vi "main.vi"() -> ()   [LabVIEW 2019]
uses:
  LabJackU3/temperature_status_LabJackU3.ctl
  MKS946/cluster_ref_MKS946.ctl
  MaxiGauge/cluster_ref_MaxiGauge.ctl
  Fridge_Valve/cluster_ref_fridge_valve.ctl
  BGA244/cluster_ref_BGA244.ctl
  TPG361/cluster_ref_TPG361.ctl
  MCC_ETC/cluster_ref_MCCETC.ctl
  MKS670/cluster_ref_MKS670.ctl
  LabJackU3/cluster_ref_LabJackU3.ctl
  ITM10/cluster_ref_ITM10.ctl
  THCD_401/cluster_ref_thcd401.ctl
  Magnet_PS/cluster_ref_MagPS.ctl
  LakeShore218/cluster_ref_LakeShore218.ctl
  RootsPumpLCW/cluster_ref_RootsPumpLCW.ctl
  THCD_400/thcd_controls/variable_reference.ctl
panel:
  out "level_fridge_LHe":dbl(slide) caption="%" scale=0.0..45.0 scale format="%#.1f"
  out "level_fridge_LN2":dbl(slide) caption="%" scale=0.0..100.0 scale format="%#.1f"
  out "MCCETC02_T7":dbl caption="Sep. Line" format="%.1f"
  in  "open_RPLCW":bool caption="open_THCD_400"
  out "RPLCW_WFS1":dbl caption="WFS1" format="%.1f"
  out "RPLCW_M4":dbl caption="M4" format="%.1f"
  out "RPLCW_M3":dbl caption="M3" format="%.1f"
  out "PRLCW_M2":dbl caption="M2" format="%.1f"
  out "RPLCW_M1":dbl caption="M1" format="%.1f"
  out "RPLCW_status":bool
  in  "open_LS218_02":bool caption="open_THCD_400"
  out "LS218_02_T7":dbl format="%.1f"
  out "LS218_02_T6":dbl format="%.1f"
  out "LS218_02_T5":dbl format="%.1f"
  out "LS218_02_T4":dbl format="%.1f"
  out "LS218_02_T3":dbl caption="W" format="%.1f"
  out "LS218_02_T2":dbl format="%.1f"
  out "LS218_02_T1":dbl caption="W" format="%.1f"
  out "LS218_02_status":bool
  out "Nose LHe Level":dbl(slide) caption="%" scale=0.0..100.0 scale format="%#_1f"
  in  "open_MagPS":bool caption="open_THCD_400"
  out "MagPS_status":bool
  out "LS218_01_T8":dbl caption="W" format="%.1f"
  out "LS218_01_T7":dbl caption="W" format="%.1f"
  out "LS218_01_T6":dbl caption="W" format="%.1f"
  out "LS218_01_T5":dbl caption="W" format="%.1f"
  out "LS218_01_T4":dbl caption="W" format="%.1f"
  out "LS218_01_T3":dbl caption="W" format="%.1f"
  out "LS218_01_T2":dbl caption="W" format="%.1f"
  out "LS218_01_T1":dbl caption="W" format="%.1f"
  out "THCD401_status":bool
  out "FC1":dbl format="%.2f"
  out "FC2":dbl format="%.2f"
  out "FM1":dbl format="%.2f"
  in  "open_THCD_401":bool caption="open_THCD_400"
  out "MCCETC03_T5":dbl format="%.1f"
  out "MCCETC03_T4":dbl format="%.1f"
  in  "open_ITM10":bool caption="open_THCD_400"
  out "T_Coil_B":dbl caption="Coil B" format="%.1f"
  out "T_Coil_T":dbl caption="Coil T" format="%.1f"
  out "T_Tank_B":dbl caption="Tank B" format="%.1f"
  out "T_Tank_T":dbl caption="Tank T" format="%.1f"
  out "ITM10_status":bool
  out "MG5":dbl caption="psi" format="%.2f"
  in  "open_LJU3_TC":bool caption="open_THCD_400"
  out "LJU3_T_status":T1=enum."UNKNOWN" caption="QT Comp. LCW Temp."
  out "LJU3_TC_status":bool
  out "MKS670_100_status":bool
  out "p_mks670_100":dbl caption="Torr"
  in  "open_LS218_01":bool caption="open_THCD_400"
  out "LS218_01_status":bool
  in  "open_MCCETC03":bool caption="open_THCD_400"
  out "MCCETC03_T3":dbl caption="T3" format="%.1f"
  out "MCCETC03_T2":dbl caption="T2" format="%.1f"
  out "MCCETC03_T1":dbl caption="T1" format="%.1f"
  out "MCCETC03_T0":dbl caption="T0" format="%.1f"
  out "MCCETC03_status":bool
  in  "open_MCCETC01":bool caption="open_THCD_400"
  out "MCCETC01_T7":dbl caption="DR" format="%.1f"
  out "MCCETC01_T6":dbl caption="DL" format="%.1f"
  out "MCCETC01_T5":dbl caption="DB" format="%.1f"
  out "MCCETC01_T4":dbl caption="DT" format="%.1f"
  out "MCCETC01_T3":dbl caption="UR" format="%.1f"
  out "MCCETC01_T2":dbl caption="UL" format="%.1f"
  out "MCCETC01_T1":dbl caption="UB" format="%.1f"
  out "MCCETC01_T0":dbl caption="UT" format="%.1f"
  out "MCCETC01_status":bool
  out "MCCETC02_T6":dbl caption="Sep. Line" format="%.2f"
  out "MCCETC02_T5":dbl caption="LHe FL #2" format="%.1f"
  out "MCCETC02_T4":dbl caption="LHe FL #1" format="%.1f"
  out "MCCETC02_T3":dbl caption="LHe FL Stinger" format="%.1f"
  out "MCCETC02_T2":dbl caption="Fridge Top" format="%.1f"
  in  "open_MCCETC02":bool caption="open_THCD_400"
  out "MCCETC02_T1":dbl caption="IVC Top" format="%.2f"
  out "MCCETC02_T0":dbl caption="IVC Bottom" format="%.2f"
  out "MCCETC02_status":bool
  in  "open_TPG361":bool caption="open_THCD_400"
  out "TPG361_p":dbl caption="IVC" format="%_3e"
  out "TPG361_status":bool
  in  "open_BGA244":bool caption="open_THCD_400"
  out "Purity":dbl caption="%" format="%.2f"
  out "BGA244_status":bool
  out "MKS670_He3_status":bool
  out "MKS670_1000_status":bool
  in  "all_stop_button":bool
  in  "open_MaxiGauge":bool
  out "MG_status":bool
  out "MG4":dbl format="%_4f"
  out "MG3":dbl format="%_4f"
  out "MG2":dbl caption="Torr" format="%_4f"
  out "MG1":dbl caption="Torr" format="%_4f"
  out "Fridge_Valve_status":bool
  in  "open_Fridge_Valve":bool
  in  "open_MKS670_He3":bool
  in  "open_MKS670_100":bool
  in  "open_MKS670_1000":bool
  in  "open_THCD_400":bool
  out "THCD400_status":bool
  out "FC1_400":dbl format="%.2f"
  out "FC2_400":dbl format="%.2f"
  out "FM1_400":dbl caption="Fridge Return" format="%.2f"
  out "Bypass Valve":dbl format="%_3f"
  out "P2":dbl caption="Root Exhaust" format="%.2f"
  out "He3 Vapor Pressure":dbl
  out "MKS946_status":bool
  out "p_mks670_1000":dbl caption="Torr"
  out "Run-Valve":dbl format="%_3f"
  in  "open_MKS946":bool
  out "P1":dbl caption="QT Manifold" format="%.2f"
  in  "STOP VI":bool
  # "THCD-400"
  # "Click a reading and stay for 1 sec to find its controller name."
  # "Fridge Temperatures"
  # "GPM"
  # "Microwave System"
  # "psi"
  # "°C"
  # "L/m"
  # "psi"
  # "Turns"
  # "L/m"
  # "L/m"
  # "°C"
  # "°C"
  # "Controller"
  # "Status"
  # "Sub Panel"
  # "Torr"
  # "Torr"
  # "MKS 670 / 1000"
  # "Cooldown-Line Temp."
  # "°C"
  # "MKS 670 /   100"
  # "K"
  # "MKS 670 / He3"
  # "Turns"
  # "MKS 946"
  # "THCD-401"
  # "°C"
  # "MaxiGauge"
  # "K"
  # "Fridge Valve"
  # "°C"
  # "Target-Cup\nTemperatures"
  # "°C"
  # "K"
  # "BGA244"
  # "TPG361"
  # "°C"
  # "K"
  # "ITM10"
  # "Torr"
  # "W"
  # "MCC E-TC #01"
  # "K"
  # "MCC E-TC #02"
  # "°C"
  # "Torr"
  # "%"
  # "MCC E-TC #03"
  # "K"
  # "LakeShore218 #01"
  # "K"
  # "LakeShore218 #02"
  # "%"
  # "°C"
  # "Roots-Pump LCW"
  # "Magnet Surface Temperature"
  # "LabJack U3 TC"
  # "K"
  # "Magnet PS"
  # "K"
  # "Schematic Version 7.0"
  # "Cryo Control Panel"
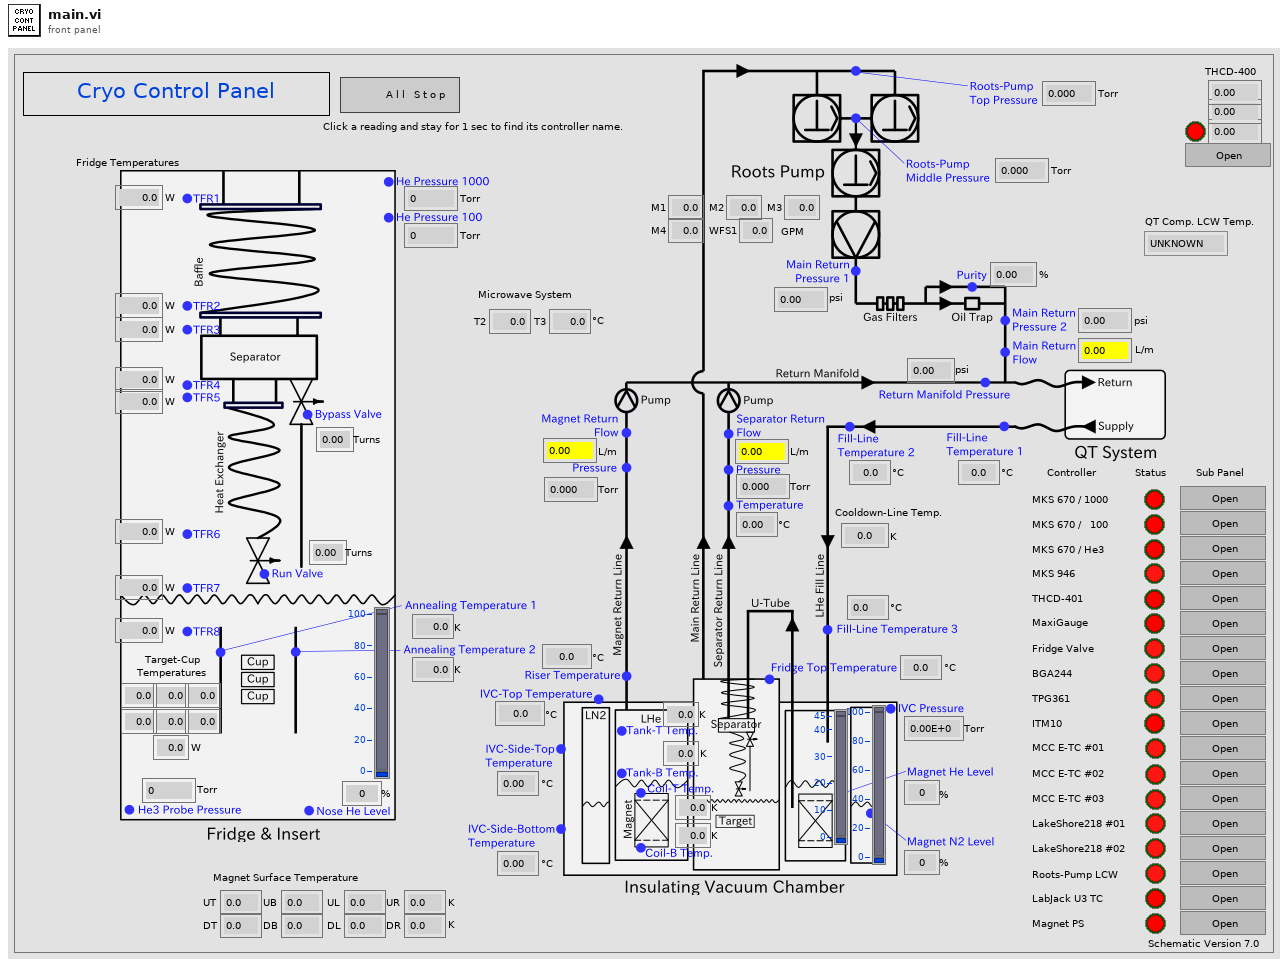
[diagram p1: front panel]
types:
  T1 = typedef "temperature_status_LabJackU3.ctl" = enum16{"OK", "UNKNOWN", "WARNING", "ERROR"}
  T2 = typedef "cluster_ref_RootsPumpLCW.ctl" = cluster{"Status":refnum<vi>, "M1":refnum<vi>, "M2":refnum<vi>, "M3":refnum<vi>, "M4":refnum<vi>, "WFS1":refnum<vi>}
  T3 = typedef "cluster_ref_LakeShore218.ctl" = cluster{"Status":refnum<vi>, "value_array":refnum<vi>, "T":refnum<vi>[]}
  T4 = typedef "cluster_ref_MagPS.ctl" = cluster{"Status":refnum<vi>, "level_LHe":refnum<vi>, "level_LN2":refnum<vi>}
  T5 = typedef "cluster_ref_thcd401.ctl" = cluster{"Status":refnum<vi>, "FM1":refnum<vi>, "FC1":refnum<vi>, "FC2":refnum<vi>}
  T6 = typedef "cluster_ref_ITM10.ctl" = cluster{"Status":refnum<vi>, "T":refnum<vi>[]}
  T7 = typedef "cluster_ref_LabJackU3.ctl" = cluster{"Status":refnum<vi>, "Temperature":refnum<vi>}
  T8 = typedef "cluster_ref_MKS670.ctl" = cluster{"status":refnum<vi>, "PR":refnum<vi>}
  T9 = typedef "cluster_ref_MCCETC.ctl" = cluster{"Status":refnum<vi>, "T":refnum<vi>[]}
  T10 = typedef "cluster_ref_TPG361.ctl" = cluster{"Status":refnum<vi>, "PR1":refnum<vi>}
  T11 = typedef "cluster_ref_BGA244.ctl" = cluster{"Status":refnum<vi>, "purity":refnum<vi>}
  T12 = typedef "cluster_ref_fridge_valve.ctl" = cluster{"Status":refnum<vi>, "RVO":refnum<vi>, "BVO":refnum<vi>, "He Level":refnum<vi>}
  T13 = typedef "cluster_ref_MaxiGauge.ctl" = cluster{"status":refnum<vi>, "MG1":refnum<vi>, "MG2":refnum<vi>, "MG3":refnum<vi>, "MG4":refnum<vi>, "MG5":refnum<vi>}
  T14 = typedef "cluster_ref_MKS946.ctl" = cluster{"Status":refnum<vi>, "PR1":refnum<vi>, "PR2":refnum<vi>}
  T15 = typedef "variable_reference.ctl" = cluster{"Status":refnum<vi>, "FM1":refnum<vi>, "FC1":refnum<vi>, "FC2":refnum<vi>}
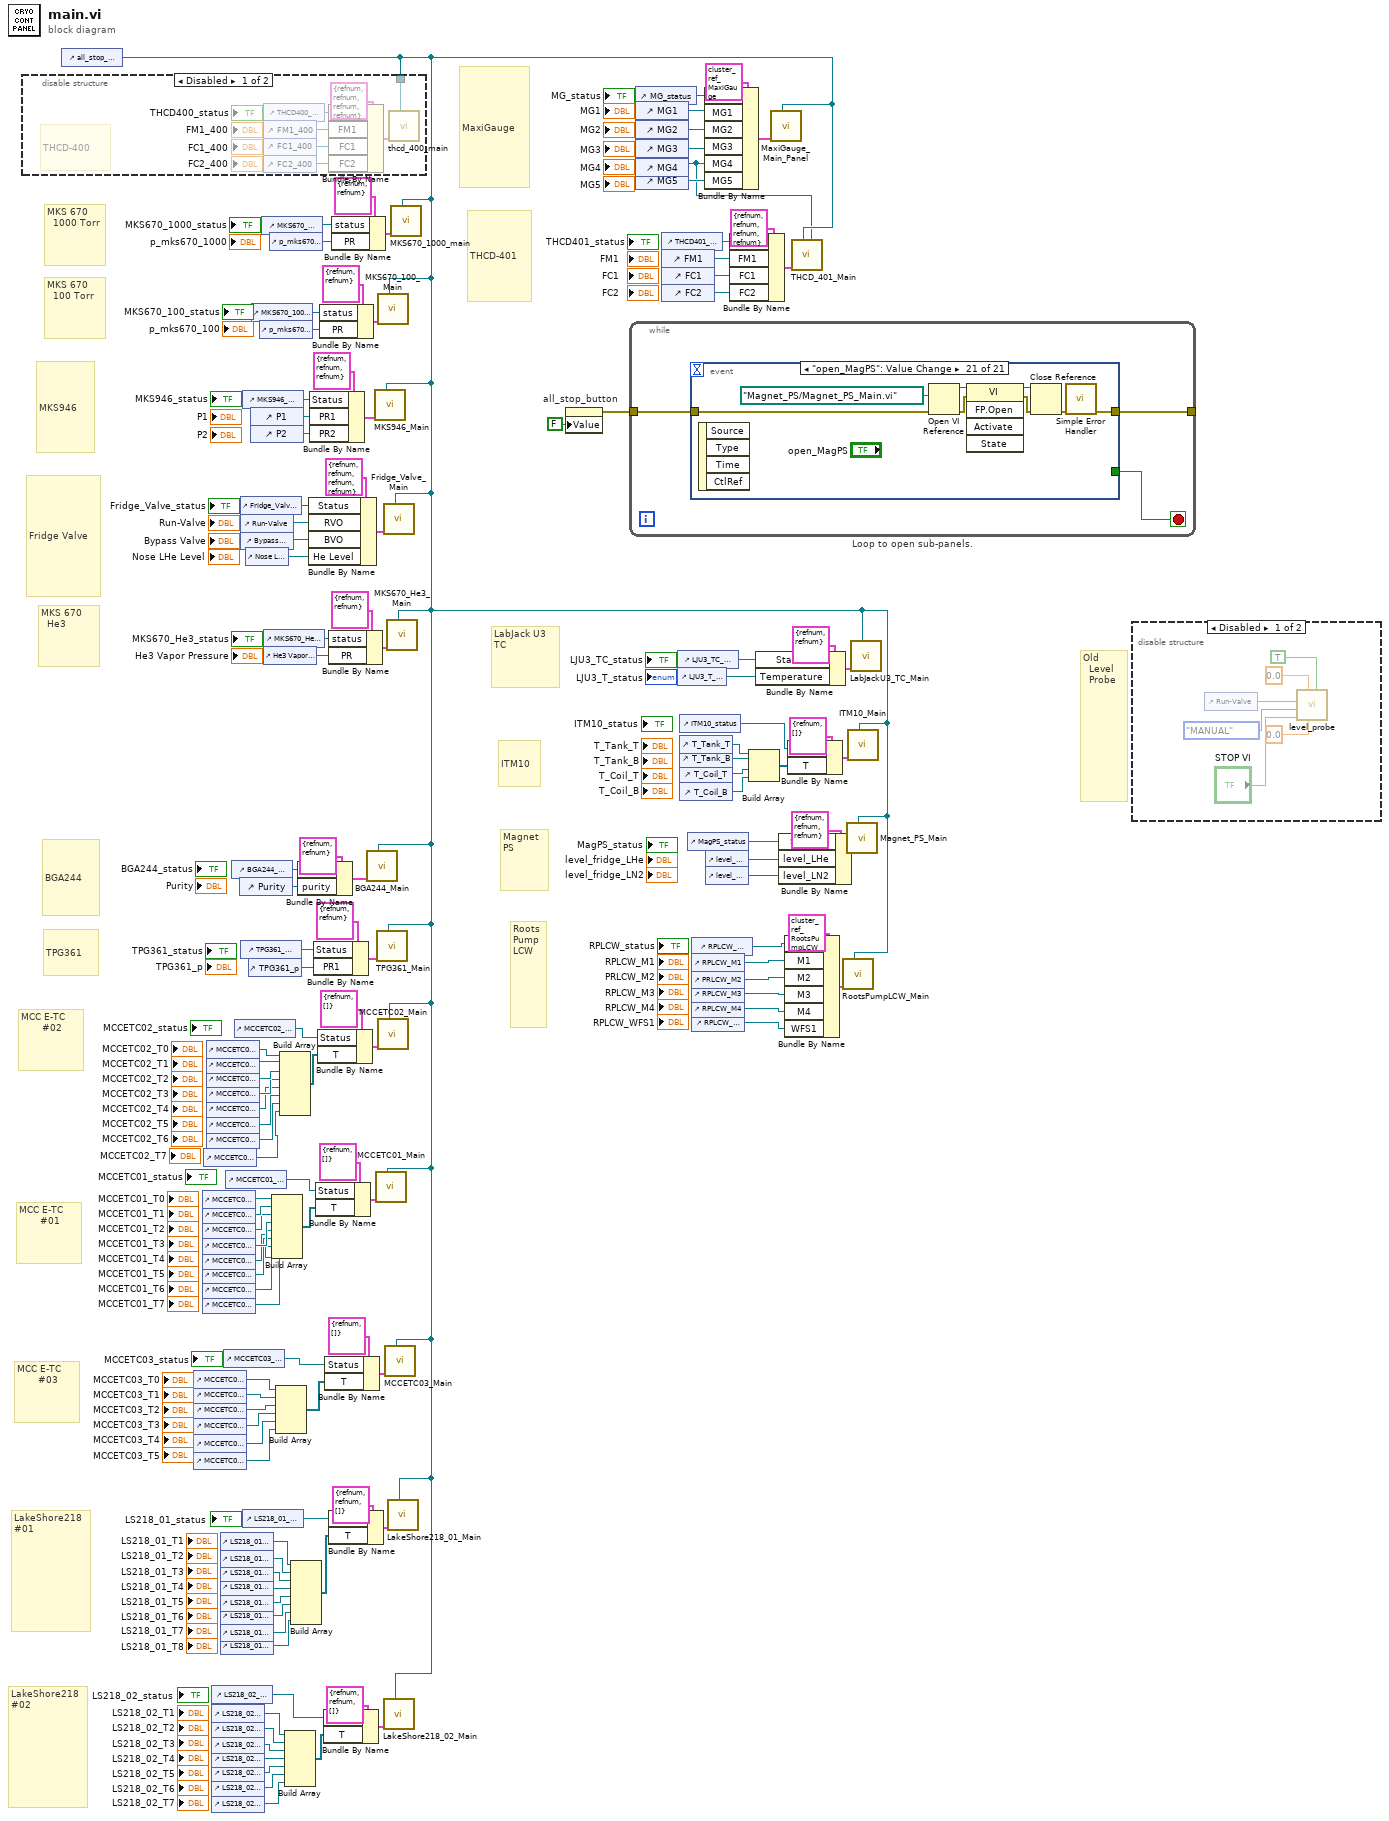
[diagram p0: block diagram]
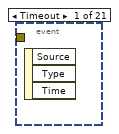
[diagram p3: hidden frame]
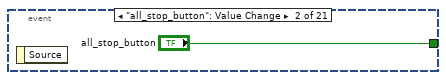
[diagram p4: hidden frame]
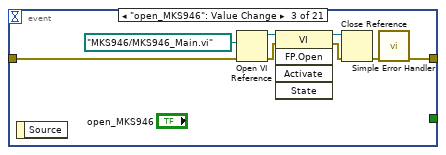
[diagram p5: hidden frame]
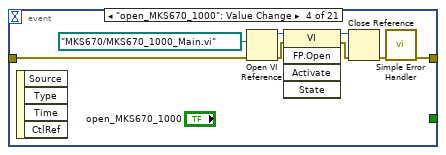
[diagram p6: hidden frame]
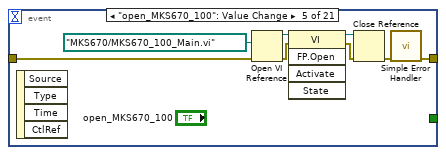
[diagram p7: hidden frame]
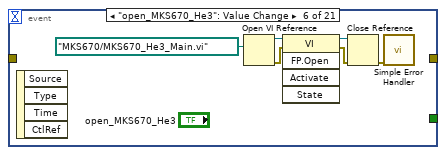
[diagram p8: hidden frame]
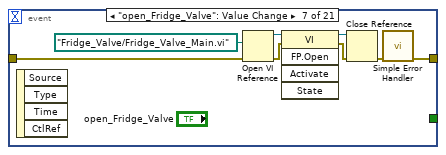
[diagram p9: hidden frame]
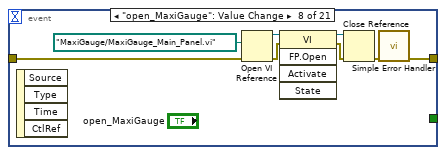
[diagram p10: hidden frame]
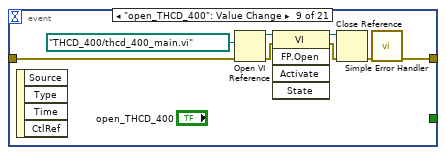
[diagram p11: hidden frame]
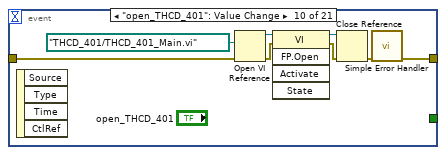
[diagram p12: hidden frame]
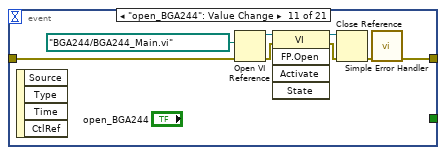
[diagram p13: hidden frame]
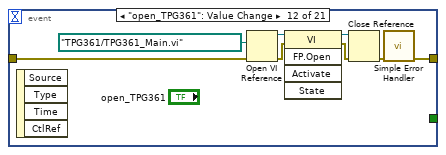
[diagram p14: hidden frame]
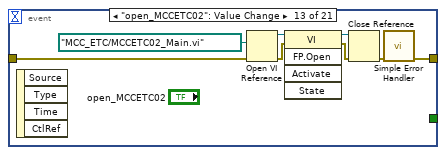
[diagram p15: hidden frame]
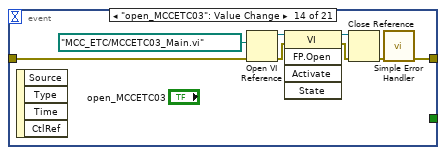
[diagram p16: hidden frame]
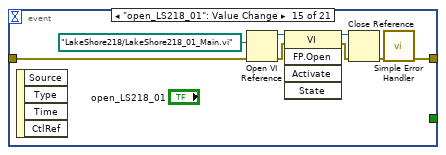
[diagram p17: hidden frame]
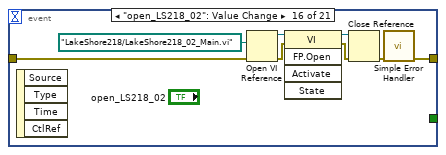
[diagram p18: hidden frame]
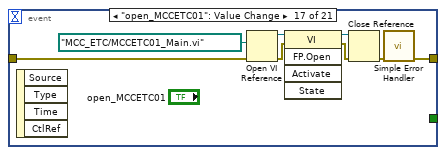
[diagram p19: hidden frame]
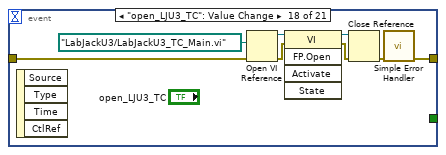
[diagram p20: hidden frame]
diagram:
  # "THCD-401"
  # "Roots\nPump\nLCW"
  # "LakeShore218\n#02"
  # "Magnet\nPS"
  # "ITM10"
  # "LabJack U3 \nTC"
  # "MKS 670  \n  100 Torr"
  # "LakeShore218\n#01"
  # "MCC E-TC\n       #03"
  # "MCC E-TC\n       #01"
  # "MCC E-TC\n       #02"
  # "TPG361"
  # "BGA244"
  # "Fridge Valve"
  # "MKS 670  \n  He3"
  # "MaxiGauge"
  # "MKS 670  \n  1000 Torr"
  # "Old\n  Level  \n  Probe"
  # "MKS946"
  n1 = control-ref of="all_stop_button"() -> (w4:refnum<vi>)
  n2 = disable-structure shown="Disabled" {
    disable-tunnel: w4 -> [w131 _]
    frame Disabled {
      # "THCD-400"
      n3 = control-ref of="THCD400_status"() -> (w136:refnum<vi>)
      n4 = control-ref of="FM1_400"() -> (w135:refnum<vi>)
      n5 = control-ref of="FC1_400"() -> (w134:refnum<vi>)
      n6 = control-ref of="FC2_400"() -> (w133:refnum<vi>)
      n7 = Bundle By Name(cluster=T15 {"Status"=refnum, "FM1"=refnum, "FC1"=refnum, "FC2"=refnum} ("variable_ref"), "Status"=w136, "FM1"=w135, "FC1"=w134, "FC2"=w133) -> (w132:T15)
      n8 = call "thcd_400_main.vi"("stop_external"=w131, "variable_ref"=w132) -> ()  [unwired: 10 in]
    }
    frame Enabled {
    }
  }
  n9 = control-ref of="MCCETC03_T0"() -> (w76:refnum<vi>)
  n10 = control-ref of="MCCETC03_T1"() -> (w77:refnum<vi>)
  n11 = control-ref of="MCCETC03_T2"() -> (w75:refnum<vi>)
  n12 = control-ref of="MCCETC03_T3"() -> (w74:refnum<vi>)
  n13 = control-ref of="MCCETC03_T4"() -> (w44:refnum<vi>)
  n14 = control-ref of="MCCETC03_T5"() -> (w43:refnum<vi>)
  n15 = control-ref of="MCCETC01_T0"() -> (w89:refnum<vi>)
  n16 = control-ref of="MCCETC01_T1"() -> (w88:refnum<vi>)
  n17 = control-ref of="MCCETC01_T2"() -> (w87:refnum<vi>)
  n18 = control-ref of="MCCETC01_T3"() -> (w86:refnum<vi>)
  n19 = control-ref of="MCCETC01_T4"() -> (w85:refnum<vi>)
  n20 = control-ref of="MCCETC01_T5"() -> (w84:refnum<vi>)
  n21 = control-ref of="MCCETC01_T6"() -> (w83:refnum<vi>)
  n22 = control-ref of="MCCETC01_T7"() -> (w82:refnum<vi>)
  n23 = control-ref of="MCCETC02_T7"() -> (w5:refnum<vi>)
  n24 = control-ref of="MCCETC02_T0"() -> (w101:refnum<vi>)
  n25 = control-ref of="MCCETC02_T1"() -> (w100:refnum<vi>)
  n26 = control-ref of="MCCETC02_T2"() -> (w98:refnum<vi>)
  n27 = control-ref of="MCCETC02_T3"() -> (w97:refnum<vi>)
  n28 = control-ref of="MCCETC02_T4"() -> (w96:refnum<vi>)
  n29 = control-ref of="MCCETC02_T5"() -> (w95:refnum<vi>)
  n30 = control-ref of="MCCETC02_T6"() -> (w94:refnum<vi>)
  n31 = control-ref of="LS218_02_status"() -> (w22:refnum<vi>)
  n32 = control-ref of="LS218_02_T1"() -> (w18:refnum<vi>)
  n33 = control-ref of="LS218_02_T2"() -> (w19:refnum<vi>)
  n34 = control-ref of="LS218_02_T3"() -> (w20:refnum<vi>)
  n35 = control-ref of="LS218_02_T4"() -> (w21:refnum<vi>)
  n36 = control-ref of="LS218_02_T5"() -> (w17:refnum<vi>)
  n37 = control-ref of="LS218_02_T6"() -> (w16:refnum<vi>)
  n38 = control-ref of="LS218_02_T7"() -> (w15:refnum<vi>)
  n39 = control-ref of="LS218_01_T1"() -> (w33:refnum<vi>)
  n40 = control-ref of="LS218_01_T2"() -> (w34:refnum<vi>)
  n41 = control-ref of="LS218_01_T3"() -> (w35:refnum<vi>)
  n42 = control-ref of="LS218_01_T4"() -> (w36:refnum<vi>)
  n43 = control-ref of="LS218_01_T5"() -> (w32:refnum<vi>)
  n44 = control-ref of="LS218_01_T6"() -> (w29:refnum<vi>)
  n45 = control-ref of="LS218_01_T7"() -> (w31:refnum<vi>)
  n46 = control-ref of="LS218_01_T8"() -> (w30:refnum<vi>)
  n47 = control-ref of="MCCETC03_status"() -> (w79:refnum<vi>)
  n48 = control-ref of="MCCETC01_status"() -> (w91:refnum<vi>)
  n49 = control-ref of="BGA244_status"() -> (w110:refnum<vi>)
  n50 = control-ref of="MCCETC02_status"() -> (w102:refnum<vi>)
  n51 = control-ref of="Purity"() -> (w109:refnum<vi>)
  n52 = control-ref of="Fridge_Valve_status"() -> (w117:refnum<vi>)
  n53 = control-ref of="Run-Valve"() -> (w115:refnum<vi>)
  n54 = control-ref of="Bypass Valve"() -> (w114:refnum<vi>)
  n55 = control-ref of="TPG361_status"() -> (w106:refnum<vi>)
  n56 = control-ref of="MKS946_status"() -> (w126:refnum<vi>)
  n57 = control-ref of="LS218_01_status"() -> (w71:refnum<vi>)
  n58 = control-ref of="Nose LHe Level"() -> (w62:refnum<vi>)
  n59 = control-ref of="TPG361_p"() -> (w105:refnum<vi>)
  n60 = control-ref of="P1"() -> (w127:refnum<vi>)
  n61 = control-ref of="P2"() -> (w128:refnum<vi>)
  n62 = control-ref of="MKS670_100_status"() -> (w68:refnum<vi>)
  n63 = control-ref of="p_mks670_100"() -> (w67:refnum<vi>)
  n64 = control-ref of="MKS670_1000_status"() -> (w64:refnum<vi>)
  n65 = control-ref of="MKS670_He3_status"() -> (w59:refnum<vi>)
  n66 = control-ref of="He3 Vapor Pressure"() -> (w58:refnum<vi>)
  n67 = control-ref of="p_mks670_1000"() -> (w63:refnum<vi>)
  n68 = Build Array(w89, w88, w87, w86, w85, w84, w83, w82) -> (w90:refnum<vi>[])
  n69 = Build Array(w76, w77, w75, w74, w44, w43) -> (w78:refnum<vi>[])
  n70 = Build Array(w101, w100, w98, w97, w96, w95, w94, w5) -> (w99:refnum<vi>[])
  n71 = Build Array(w18, w19, w20, w21, w17, w16, w15) -> (w14:refnum<vi>[])
  n72 = Build Array(w33, w34, w35, w36, w32, w29, w31, w30) -> (w28:refnum<vi>[])
  n73 = Bundle By Name(cluster=T11 {"Status"=refnum, "purity"=refnum} ("cluster_ref_BGA244"), "Status"=w110, "purity"=w109) -> (w111:T11)
  n74 = Bundle By Name(cluster=T12 {"Status"=refnum, "RVO"=refnum, "BVO"=refnum, "He Level"=refnum} ("input cluster"), "Status"=w117, "RVO"=w115, "BVO"=w114, "He Level"=w62) -> (w113:T12)
  n75 = Bundle By Name(cluster=T14 {"Status"=refnum, "PR1"=refnum, "PR2"=refnum} ("input cluster"), "Status"=w126, "PR1"=w127, "PR2"=w128) -> (w129:T14)
  n76 = Bundle By Name(cluster=T10 {"Status"=refnum, "PR1"=refnum} ("cluster_ref_TPG361"), "Status"=w106, "PR1"=w105) -> (w107:T10)
  n77 = Bundle By Name(cluster=T9 {"Status"=refnum, "T"=[]} ("input cluster"), "Status"=w91, "T"=w90) -> (w93:T9)
  n78 = Bundle By Name(cluster=T9 {"Status"=refnum, "T"=[]} ("input cluster"), "Status"=w102, "T"=w99) -> (w104:T9)
  n79 = Bundle By Name(cluster=T8 {"status"=refnum, "PR"=refnum} ("input cluster"), "status"=w68, "PR"=w67) -> (w70:T8)
  n80 = Bundle By Name(cluster=T3 {"Status"=refnum, "value_array"=refnum, "T"=[]} ("cluster_ref"), "Status"=w22, "T"=w14) -> (w23:T3)
  n81 = Bundle By Name(cluster=T9 {"Status"=refnum, "T"=[]} ("input cluster"), "Status"=w79, "T"=w78) -> (w80:T9)
  n82 = Bundle By Name(cluster=T8 {"status"=refnum, "PR"=refnum} ("input cluster"), "status"=w59, "PR"=w58) -> (w61:T8)
  n83 = Bundle By Name(cluster=T3 {"Status"=refnum, "value_array"=refnum, "T"=[]} ("cluster_ref"), "Status"=w71, "T"=w28) -> (w72:T3)
  n84 = Bundle By Name(cluster=T8 {"status"=refnum, "PR"=refnum} ("input cluster"), "status"=w64, "PR"=w63) -> (w66:T8)
  n85 = call "BGA244_Main.vi"("stop_external"=w4, "cluster_ref_BGA244"=w111) -> ()  [unwired: 10 in]
  n86 = call "MKS946_Main.vi"("stop_external"=w4, "input cluster"=w129) -> ()  [unwired: 10 in]
  n87 = call "MCCETC01_Main.vi"("stop_external"=w4, "input cluster"=w93) -> ()  [unwired: 10 in]
  n88 = call "TPG361_Main.vi"("stop_external"=w4, "cluster_ref_TPG361"=w107) -> ()  [unwired: 10 in]
  n89 = call "MKS670_100_Main.vi"("stop_external"=w4, "input cluster"=w70) -> ()  [unwired: 10 in]
  n90 = call "MCCETC02_Main.vi"("stop_external"=w4, "input cluster"=w104) -> ()  [unwired: 10 in]
  n91 = call "Fridge_Valve_Main.vi"("stop_external"=w4, "cluster_ref_fridge_valve"=w113) -> ()  [unwired: 10 in]
  n92 = call "LakeShore218_02_Main.vi"("stop_external"=w4, "cluster_ref"=w23) -> ()  [unwired: 10 in]
  n93 = call "MCCETC03_Main.vi"("stop_external"=w4, "input cluster"=w80) -> ()  [unwired: 10 in]
  n94 = call "MKS670_He3_Main.vi"("stop_external"=w4, "input cluster"=w61) -> ()  [unwired: 10 in]
  n95 = call "LakeShore218_01_Main.vi"("stop_external"=w4, "cluster_ref"=w72) -> ()  [unwired: 10 in]
  n96 = call "MKS670_1000_main.vi"("stop_external"=w4, "input cluster"=w66) -> ()  [unwired: 10 in]
  n97 = property on="all_stop_button" class="Bool (strict)"("Value"=FALSE ("all_stop_button")) -> (error out=w124:errorcluster)  [unwired: 2 in, 1 out]
  n98 = while "Loop to open sub-panels." {
    tunnel: w124 -> [w139]
    tunnel: [w138] -> _
    stop <- w140 stop-if-true
    n99 = event shown="[20] \"open_MagPS\": Value Change" {
      selector: _ -> [_ _ _ _ _ _ _ _ _ _ _ _ _ _ _ _ _ _ _ _ _]
      dyn-events: _ -> [_ _ _ _ _ _ _ _ _ _ _ _ _ _ _ _ _ _ _ _ _]
      timeout: _ -> [_ _ _ _ _ _ _ _ _ _ _ _ _ _ _ _ _ _ _ _ _]
      tunnel: [_ "all_stop_button" _ _ _ _ _ _ _ _ _ _ _ _ _ _ _ _ _ _ _] -> w140
      tunnel: w139 -> [_ _ w143 w151 w159 _ w173 w181 w189 w197 w205 w213 w221 w229 w237 w245 w253 w261 w269 w277 w285]
      tunnel: [_ _ w142 w150 w158 _ w172 w180 w188 w196 w204 w212 w220 w228 w236 w244 w252 w260 w268 w276 w284] -> w138
      event Timeout {
        n100 = event-data() -> ()  [unwired: 1 in, 3 out]
      }
      event "all_stop_button": Value Change {
        n101 = event-data() -> ()  [unwired: 1 in, 1 out]
      }
      event "open_MKS946": Value Change {
        n102 = event-data() -> ()  [unwired: 1 in, 1 out]
        n103 = Open VI Reference(vi path=path "MKS946/MKS946_Main.vi", error in (no error)=w143) -> (vi reference=w145:refnum<vi>, error out=w146:errorcluster)  [unwired: 4 in]
        n104 = invoke class="VI" method="FP.Open"(reference=w145, error in=w146) -> (reference out=w148:refnum<vi>, error out=w149:errorcluster)  [unwired: 3 in, 3 out]
        n105 = Close Reference(reference=w148, error in (no error)=w149) -> (error out=w147:errorcluster)
        n106 = call <vilib>:"Simple Error Handler.vi"("error in (no error)"=w147) -> ("error out"=w142:errorcluster)  [unwired: 4 in, 4 out]
      }
      event "open_MKS670_1000": Value Change {
        n107 = event-data() -> ()  [unwired: 1 in, 4 out]
        n108 = Open VI Reference(vi path=path "MKS670/MKS670_1000_Main.vi", error in (no error)=w151) -> (vi reference=w153:refnum<vi>, error out=w154:errorcluster)  [unwired: 4 in]
        n109 = invoke class="VI" method="FP.Open"(reference=w153, error in=w154) -> (reference out=w156:refnum<vi>, error out=w157:errorcluster)  [unwired: 3 in, 3 out]
        n110 = Close Reference(reference=w156, error in (no error)=w157) -> (error out=w155:errorcluster)
        n111 = call <vilib>:"Simple Error Handler.vi"("error in (no error)"=w155) -> ("error out"=w150:errorcluster)  [unwired: 4 in, 4 out]
      }
      event "open_MKS670_100": Value Change {
        n112 = event-data() -> ()  [unwired: 1 in, 4 out]
        n113 = Open VI Reference(vi path=path "MKS670/MKS670_100_Main.vi", error in (no error)=w159) -> (vi reference=w165:refnum<vi>, error out=w164:errorcluster)  [unwired: 4 in]
        n114 = invoke class="VI" method="FP.Open"(reference=w165, error in=w164) -> (reference out=w162:refnum<vi>, error out=w161:errorcluster)  [unwired: 3 in, 3 out]
        n115 = Close Reference(reference=w162, error in (no error)=w161) -> (error out=w163:errorcluster)
        n116 = call <vilib>:"Simple Error Handler.vi"("error in (no error)"=w163) -> ("error out"=w158:errorcluster)  [unwired: 4 in, 4 out]
      }
      event "open_MKS670_He3": Value Change {
        n117 = event-data() -> ()  [unwired: 1 in, 4 out]
        n118 = Open VI Reference(vi path=path "MKS670/MKS670_He3_Main.vi") -> (vi reference=w170:refnum<vi>, error out=w169:errorcluster)  [unwired: 5 in]
        n119 = invoke class="VI" method="FP.Open"(reference=w170, error in=w169) -> (reference out=w167:refnum<vi>, error out=w166:errorcluster)  [unwired: 3 in, 3 out]
        n120 = Close Reference(reference=w167, error in (no error)=w166) -> (error out=w168:errorcluster)
        n121 = call <vilib>:"Simple Error Handler.vi"("error in (no error)"=w168) -> ()  [unwired: 4 in, 5 out]
      }
      event "open_Fridge_Valve": Value Change {
        n122 = event-data() -> ()  [unwired: 1 in, 4 out]
        n123 = Open VI Reference(vi path=path "Fridge_Valve/Fridge_Valve_Main.vi", error in (no error)=w173) -> (vi reference=w178:refnum<vi>, error out=w177:errorcluster)  [unwired: 4 in]
        n124 = invoke class="VI" method="FP.Open"(reference=w178, error in=w177) -> (reference out=w175:refnum<vi>, error out=w174:errorcluster)  [unwired: 3 in, 3 out]
        n125 = Close Reference(reference=w175, error in (no error)=w174) -> (error out=w176:errorcluster)
        n126 = call <vilib>:"Simple Error Handler.vi"("error in (no error)"=w176) -> ("error out"=w172:errorcluster)  [unwired: 4 in, 4 out]
      }
      event "open_MaxiGauge": Value Change {
        n127 = event-data() -> ()  [unwired: 1 in, 4 out]
        n128 = Open VI Reference(vi path=path "MaxiGauge/MaxiGauge_Main_Panel.vi", error in (no error)=w181) -> (vi reference=w186:refnum<vi>, error out=w185:errorcluster)  [unwired: 4 in]
        n129 = invoke class="VI" method="FP.Open"(reference=w186, error in=w185) -> (reference out=w183:refnum<vi>, error out=w182:errorcluster)  [unwired: 3 in, 3 out]
        n130 = Close Reference(reference=w183, error in (no error)=w182) -> (error out=w184:errorcluster)
        n131 = call <vilib>:"Simple Error Handler.vi"("error in (no error)"=w184) -> ("error out"=w180:errorcluster)  [unwired: 4 in, 4 out]
      }
      event "open_THCD_400": Value Change {
        n132 = event-data() -> ()  [unwired: 1 in, 4 out]
        n133 = Open VI Reference(vi path=path "THCD_400/thcd_400_main.vi", error in (no error)=w189) -> (vi reference=w191:refnum<vi>, error out=w192:errorcluster)  [unwired: 4 in]
        n134 = invoke class="VI" method="FP.Open"(reference=w191, error in=w192) -> (reference out=w194:refnum<vi>, error out=w195:errorcluster)  [unwired: 3 in, 3 out]
        n135 = Close Reference(reference=w194, error in (no error)=w195) -> (error out=w193:errorcluster)
        n136 = call <vilib>:"Simple Error Handler.vi"("error in (no error)"=w193) -> ("error out"=w188:errorcluster)  [unwired: 4 in, 4 out]
      }
      event "open_THCD_401": Value Change {
        n137 = event-data() -> ()  [unwired: 1 in, 4 out]
        n138 = Open VI Reference(vi path=path "THCD_401/THCD_401_Main.vi", error in (no error)=w197) -> (vi reference=w199:refnum<vi>, error out=w200:errorcluster)  [unwired: 4 in]
        n139 = invoke class="VI" method="FP.Open"(reference=w199, error in=w200) -> (reference out=w202:refnum<vi>, error out=w203:errorcluster)  [unwired: 3 in, 3 out]
        n140 = Close Reference(reference=w202, error in (no error)=w203) -> (error out=w201:errorcluster)
        n141 = call <vilib>:"Simple Error Handler.vi"("error in (no error)"=w201) -> ("error out"=w196:errorcluster)  [unwired: 4 in, 4 out]
      }
      event "open_BGA244": Value Change {
        n142 = event-data() -> ()  [unwired: 1 in, 4 out]
        n143 = Open VI Reference(vi path=path "BGA244/BGA244_Main.vi", error in (no error)=w205) -> (vi reference=w207:refnum<vi>, error out=w208:errorcluster)  [unwired: 4 in]
        n144 = invoke class="VI" method="FP.Open"(reference=w207, error in=w208) -> (reference out=w210:refnum<vi>, error out=w211:errorcluster)  [unwired: 3 in, 3 out]
        n145 = Close Reference(reference=w210, error in (no error)=w211) -> (error out=w209:errorcluster)
        n146 = call <vilib>:"Simple Error Handler.vi"("error in (no error)"=w209) -> ("error out"=w204:errorcluster)  [unwired: 4 in, 4 out]
      }
      event "open_TPG361": Value Change {
        n147 = event-data() -> ()  [unwired: 1 in, 4 out]
        n148 = Open VI Reference(vi path=path "TPG361/TPG361_Main.vi", error in (no error)=w213) -> (vi reference=w215:refnum<vi>, error out=w216:errorcluster)  [unwired: 4 in]
        n149 = invoke class="VI" method="FP.Open"(reference=w215, error in=w216) -> (reference out=w218:refnum<vi>, error out=w219:errorcluster)  [unwired: 3 in, 3 out]
        n150 = Close Reference(reference=w218, error in (no error)=w219) -> (error out=w217:errorcluster)
        n151 = call <vilib>:"Simple Error Handler.vi"("error in (no error)"=w217) -> ("error out"=w212:errorcluster)  [unwired: 4 in, 4 out]
      }
      event "open_MCCETC02": Value Change {
        n152 = event-data() -> ()  [unwired: 1 in, 4 out]
        n153 = Open VI Reference(vi path=path "MCC_ETC/MCCETC02_Main.vi", error in (no error)=w221) -> (vi reference=w223:refnum<vi>, error out=w224:errorcluster)  [unwired: 4 in]
        n154 = invoke class="VI" method="FP.Open"(reference=w223, error in=w224) -> (reference out=w226:refnum<vi>, error out=w227:errorcluster)  [unwired: 3 in, 3 out]
        n155 = Close Reference(reference=w226, error in (no error)=w227) -> (error out=w225:errorcluster)
        n156 = call <vilib>:"Simple Error Handler.vi"("error in (no error)"=w225) -> ("error out"=w220:errorcluster)  [unwired: 4 in, 4 out]
      }
      event "open_MCCETC03": Value Change {
        n157 = event-data() -> ()  [unwired: 1 in, 4 out]
        n158 = Open VI Reference(vi path=path "MCC_ETC/MCCETC03_Main.vi", error in (no error)=w229) -> (vi reference=w231:refnum<vi>, error out=w232:errorcluster)  [unwired: 4 in]
        n159 = invoke class="VI" method="FP.Open"(reference=w231, error in=w232) -> (reference out=w234:refnum<vi>, error out=w235:errorcluster)  [unwired: 3 in, 3 out]
        n160 = Close Reference(reference=w234, error in (no error)=w235) -> (error out=w233:errorcluster)
        n161 = call <vilib>:"Simple Error Handler.vi"("error in (no error)"=w233) -> ("error out"=w228:errorcluster)  [unwired: 4 in, 4 out]
      }
      event "open_LS218_01": Value Change {
        n162 = event-data() -> ()  [unwired: 1 in, 4 out]
        n163 = Open VI Reference(vi path=path "LakeShore218/LakeShore218_01_Main.vi", error in (no error)=w237) -> (vi reference=w239:refnum<vi>, error out=w240:errorcluster)  [unwired: 4 in]
        n164 = invoke class="VI" method="FP.Open"(reference=w239, error in=w240) -> (reference out=w242:refnum<vi>, error out=w243:errorcluster)  [unwired: 3 in, 3 out]
        n165 = Close Reference(reference=w242, error in (no error)=w243) -> (error out=w241:errorcluster)
        n166 = call <vilib>:"Simple Error Handler.vi"("error in (no error)"=w241) -> ("error out"=w236:errorcluster)  [unwired: 4 in, 4 out]
      }
      event "open_LS218_02": Value Change {
        n167 = event-data() -> ()  [unwired: 1 in, 4 out]
        n168 = Open VI Reference(vi path=path "LakeShore218/LakeShore218_02_Main.vi", error in (no error)=w245) -> (vi reference=w247:refnum<vi>, error out=w248:errorcluster)  [unwired: 4 in]
        n169 = invoke class="VI" method="FP.Open"(reference=w247, error in=w248) -> (reference out=w250:refnum<vi>, error out=w251:errorcluster)  [unwired: 3 in, 3 out]
        n170 = Close Reference(reference=w250, error in (no error)=w251) -> (error out=w249:errorcluster)
        n171 = call <vilib>:"Simple Error Handler.vi"("error in (no error)"=w249) -> ("error out"=w244:errorcluster)  [unwired: 4 in, 4 out]
      }
      event "open_MCCETC01": Value Change {
        n172 = event-data() -> ()  [unwired: 1 in, 4 out]
        n173 = Open VI Reference(vi path=path "MCC_ETC/MCCETC01_Main.vi", error in (no error)=w253) -> (vi reference=w255:refnum<vi>, error out=w256:errorcluster)  [unwired: 4 in]
        n174 = invoke class="VI" method="FP.Open"(reference=w255, error in=w256) -> (reference out=w258:refnum<vi>, error out=w259:errorcluster)  [unwired: 3 in, 3 out]
        n175 = Close Reference(reference=w258, error in (no error)=w259) -> (error out=w257:errorcluster)
        n176 = call <vilib>:"Simple Error Handler.vi"("error in (no error)"=w257) -> ("error out"=w252:errorcluster)  [unwired: 4 in, 4 out]
      }
      event "open_LJU3_TC": Value Change {
        n177 = event-data() -> ()  [unwired: 1 in, 4 out]
        n178 = Open VI Reference(vi path=path "LabJackU3/LabJackU3_TC_Main.vi", error in (no error)=w261) -> (vi reference=w263:refnum<vi>, error out=w264:errorcluster)  [unwired: 4 in]
        n179 = invoke class="VI" method="FP.Open"(reference=w263, error in=w264) -> (reference out=w266:refnum<vi>, error out=w267:errorcluster)  [unwired: 3 in, 3 out]
        n180 = Close Reference(reference=w266, error in (no error)=w267) -> (error out=w265:errorcluster)
        n181 = call <vilib>:"Simple Error Handler.vi"("error in (no error)"=w265) -> ("error out"=w260:errorcluster)  [unwired: 4 in, 4 out]
      }
      event "open_RPLCW": Value Change {
        n182 = event-data() -> ()  [unwired: 1 in, 4 out]
        n183 = Open VI Reference(vi path=path "RootsPumpLCW/RootsPumpLCW_Main.vi", error in (no error)=w269) -> (vi reference=w271:refnum<vi>, error out=w272:errorcluster)  [unwired: 4 in]
        n184 = invoke class="VI" method="FP.Open"(reference=w271, error in=w272) -> (reference out=w274:refnum<vi>, error out=w275:errorcluster)  [unwired: 3 in, 3 out]
        n185 = Close Reference(reference=w274, error in (no error)=w275) -> (error out=w273:errorcluster)
        n186 = call <vilib>:"Simple Error Handler.vi"("error in (no error)"=w273) -> ("error out"=w268:errorcluster)  [unwired: 4 in, 4 out]
      }
      event "open_ITM10": Value Change {
        n187 = event-data() -> ()  [unwired: 1 in, 4 out]
        n188 = Open VI Reference(vi path=path "ITM10/ITM10_Main.vi", error in (no error)=w277) -> (vi reference=w279:refnum<vi>, error out=w280:errorcluster)  [unwired: 4 in]
        n189 = invoke class="VI" method="FP.Open"(reference=w279, error in=w280) -> (reference out=w282:refnum<vi>, error out=w283:errorcluster)  [unwired: 3 in, 3 out]
        n190 = Close Reference(reference=w282, error in (no error)=w283) -> (error out=w281:errorcluster)
        n191 = call <vilib>:"Simple Error Handler.vi"("error in (no error)"=w281) -> ("error out"=w276:errorcluster)  [unwired: 4 in, 4 out]
      }
      event "open_MagPS": Value Change {
        n192 = event-data() -> ()  [unwired: 1 in, 4 out]
        n193 = Open VI Reference(vi path=path "Magnet_PS/Magnet_PS_Main.vi", error in (no error)=w285) -> (vi reference=w287:refnum<vi>, error out=w288:errorcluster)  [unwired: 4 in]
        n194 = invoke class="VI" method="FP.Open"(reference=w287, error in=w288) -> (reference out=w290:refnum<vi>, error out=w291:errorcluster)  [unwired: 3 in, 3 out]
        n195 = Close Reference(reference=w290, error in (no error)=w291) -> (error out=w289:errorcluster)
        n196 = call <vilib>:"Simple Error Handler.vi"("error in (no error)"=w289) -> ("error out"=w284:errorcluster)  [unwired: 4 in, 4 out]
      }
    }
  }
  n197 = control-ref of="MG_status"() -> (w123:refnum<vi>)
  n198 = control-ref of="MG1"() -> (w122:refnum<vi>)
  n199 = control-ref of="MG2"() -> (w121:refnum<vi>)
  n200 = control-ref of="MG3"() -> (w120:refnum<vi>)
  n201 = control-ref of="MG4"() -> (w3:refnum<vi>)
  n202 = control-ref of="MG5"() -> (w53:refnum<vi>)
  n203 = control-ref of="THCD401_status"() -> (w40:refnum<vi>)
  n204 = control-ref of="FM1"() -> (w39:refnum<vi>)
  n205 = control-ref of="FC1"() -> (w38:refnum<vi>)
  n206 = control-ref of="FC2"() -> (w37:refnum<vi>)
  n207 = control-ref of="LJU3_TC_status"() -> (w55:refnum<vi>)
  n208 = control-ref of="LJU3_T_status"() -> (w54:refnum<vi>)
  n209 = control-ref of="ITM10_status"() -> (w50:refnum<vi>)
  n210 = control-ref of="T_Tank_T"() -> (w48:refnum<vi>)
  n211 = control-ref of="T_Tank_B"() -> (w45:refnum<vi>)
  n212 = control-ref of="T_Coil_T"() -> (w47:refnum<vi>)
  n213 = control-ref of="T_Coil_B"() -> (w46:refnum<vi>)
  n214 = control-ref of="MagPS_status"() -> (w25:refnum<vi>)
  n215 = control-ref of="RPLCW_status"() -> (w11:refnum<vi>)
  n216 = control-ref of="RPLCW_M1"() -> (w10:refnum<vi>)
  n217 = control-ref of="PRLCW_M2"() -> (w9:refnum<vi>)
  n218 = control-ref of="RPLCW_M3"() -> (w8:refnum<vi>)
  n219 = control-ref of="RPLCW_M4"() -> (w7:refnum<vi>)
  n220 = control-ref of="RPLCW_WFS1"() -> (w6:refnum<vi>)
  n221 = Bundle By Name(cluster=T13 {"status"=refnum, "MG1"=refnum, "MG2"=refnum, "MG3"=refnum, "MG4"=refnum, "MG5"=refnum} ("input cluster"), "status"=w123, "MG1"=w122, "MG2"=w121, "MG3"=w120, "MG4"=w3, "MG5"=w53) -> (w118:T13)
  n222 = control-ref of="level_fridge_LHe"() -> (w1:refnum<vi>)
  n223 = control-ref of="level_fridge_LN2"() -> (w2:refnum<vi>)
  n224 = Bundle By Name(cluster=T5 {"Status"=refnum, "FM1"=refnum, "FC1"=refnum, "FC2"=refnum} ("variable_ref"), "Status"=w40, "FM1"=w39, "FC1"=w38, "FC2"=w37) -> (w42:T5)
  n225 = Build Array(w48, w45, w47, w46) -> (w49:refnum<vi>[])
  n226 = Bundle By Name(cluster=T7 {"Status"=refnum, "Temperature"=refnum} ("cluster_ref"), "Status"=w55, "Temperature"=w54) -> (w57:T7)
  n227 = call "MaxiGauge_Main_Panel.vi"("stop_external"=w4, "input cluster"=w118) -> ()  [unwired: 10 in]
  n228 = Bundle By Name(cluster=T4 {"Status"=refnum, "level_LHe"=refnum, "level_LN2"=refnum} ("input cluster"), "Status"=w25, "level_LHe"=w1, "level_LN2"=w2) -> (w26:T4)
  n229 = Bundle By Name(cluster=T2 {"Status"=refnum, "M1"=refnum, "M2"=refnum, "M3"=refnum, "M4"=refnum, "WFS1"=refnum} ("variable_reference"), "Status"=w11, "M1"=w10, "M2"=w9, "M3"=w8, "M4"=w7, "WFS1"=w6) -> (w13:T2)
  n230 = Bundle By Name(cluster=T6 {"Status"=refnum, "T"=[]} ("input_cluster"), "Status"=w50, "T"=w49) -> (w52:T6)
  n231 = call "THCD_401_Main.vi"("ref_magnet_pres"=w3, "stop_external"=w4, "variable_ref"=w42) -> ()  [unwired: 9 in]
  n232 = call "RootsPumpLCW_Main.vi"("ref_stop_external"=w4, "variable_reference"=w13) -> ()  [unwired: 10 in]
  n233 = call "Magnet_PS_Main.vi"("ref_stop_external"=w4, "input cluster"=w26) -> ()  [unwired: 9 in, 1 out]
  n234 = call "ITM10_Main.vi"("stop_external"=w4, "input_cluster"=w52) -> ()  [unwired: 10 in]
  n235 = call "LabJackU3_TC_Main.vi"("stop_external"=w4, "cluster_ref"=w57) -> ()  [unwired: 10 in]
  n236 = disable-structure shown="Disabled" {
    frame Disabled {
      n237 = control-ref of="Run-Valve"() -> (w298:refnum<vi>)
      n238 = call "level_probe.vi"("Run VI"=TRUE, "Set # of Turns Open (Man)"=0.0, "Target Level (Auto)"=0.0, "stop"="STOP VI", "Mode"=enum32{"AUTOMATIC", "MANUAL"}."MANUAL", "position"=w298) -> ("level"=w297:refnum<vi>)  [unwired: 5 in]
    }
    frame Enabled {
    }
  }
